vi "Add MDIF Block.vi"(7 "Block Name":string="Block", 8 "error in (no error)":errorcluster, 9 "Dependent Variables":cluster{"Name":string, "Values":refnum<k24>}[](array[cluster]), 10 "Independent Variables":cluster{"Name":string, "Values":refnum<k24>}[](array[cluster]), 11 "MDIF reference in":refnum<k24>) -> (0 "error out":errorcluster, 3 "MDIF reference out":refnum<k24>)   [LabVIEW 2023, in "NI_HFNetworkAnalysis.lvlib"]
doc: "Add a MDIF block in memory for the specified MDIF file.\n\n<b>Note</b>\nUse <b>Save MDIF File.vi</b> to write all MDIF blocks in memory to the referenced MDIF file."
uses:
  NI_HFNetworkAnalysis.lvlib
  C:/srd-semi-rfcal-software/AuxTools/STSRFFixtureCharactUtility/Source/Code Modules/Fixture/Dependencies/HFNetworkAnalysis/Support Files/NACE.Utils.Data.dll
  Support Files/NACE.Utils.Data.dll
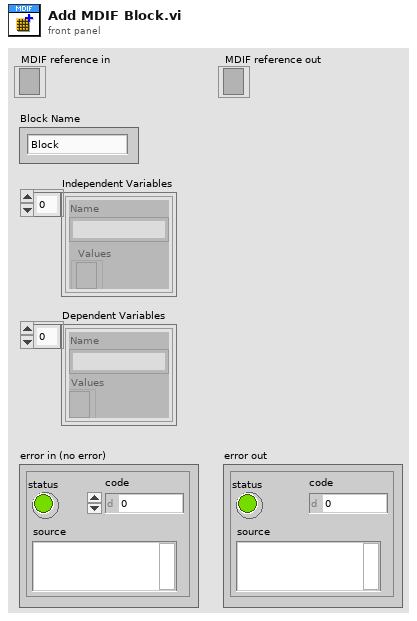
[diagram p1: front panel]
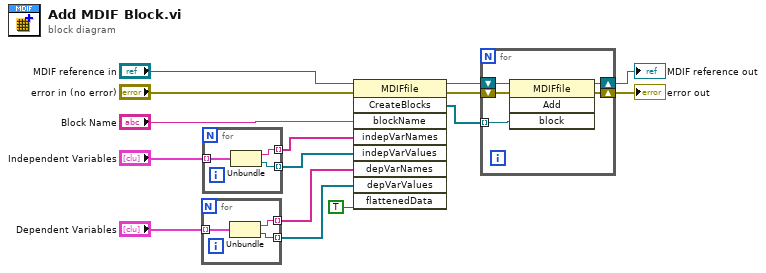
[diagram p0: block diagram]
diagram:
  n1 = for {
    tunnel: "Dependent Variables" -> [w18] mode=indexing
    tunnel: [w17] -> w3 mode=indexing
    tunnel: [w16] -> w2 mode=indexing
    n2 = Unbundle(w18) -> ("Name"=w17:string, "Values"=w16:refnum<k24>)
  }
  n3 = for {
    tunnel: "Independent Variables" -> [w21] mode=indexing
    tunnel: [w20] -> w7 mode=indexing
    tunnel: [w19] -> w6 mode=indexing
    n4 = Unbundle(w21) -> ("Name"=w20:string, "Values"=w19:refnum<k24>)
  }
  n5 = invoke class="MDIFfile" method="CreateBlocks"(reference="MDIF reference in", error in="error in (no error)", "blockName"="Block Name", "indepVarNames"=w7, "indepVarValues"=w6, "depVarNames"=w3, "depVarValues"=w2, "flattenedData"=TRUE) -> (reference out=w14:refnum<k24>, error out=w15:errorcluster, "CreateBlocks"=w13:refnum<k24>[])  [unwired: 1 in, 6 out]
  n6 = for {
    tunnel: w13 -> [w24] mode=indexing
    shift-right: [w23] -> w11
    shift-left: w15 -> [w26]
    shift-right: [w22] -> w12
    shift-left: w14 -> [w25]
    n7 = invoke class="MDIFfile" method="Add"(reference=w25, error in=w26, "block"=w24) -> (reference out=w22:refnum<k24>, error out=w23:errorcluster)  [unwired: 1 in, 2 out]
  }
  "MDIF reference out" <- w12
  "error out" <- w11
